vi "Tunnel position to Inside-Outside choice.vi"(7 "Default Placement":enum32{"Choice 1", "Choice 2"}(ring), 10 "Tunnel Position":enum16{"Left", "Top", "Right", "Bottom"}(ring), 11 "Action":T1=enum."Wire Properties") -> (3 "Placement":enum16{"Inside", "Outside"}(ring))   [LabVIEW 2023]
doc: "Choose default placement (inside/outisde) for a cluster element when a tunnel is selected. Bundling at the top/left of a structure assumes outisde, unbundling inside. Bundling at the bottom or right of a struncture is assumed inside, unbundling outside. This feels like the right choice in a majority of cases."
uses:
  controls/action enum.ctl
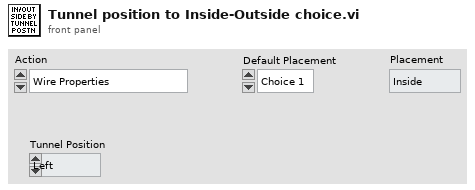
[diagram p1: front panel]
types:
  T1 = typedef "action enum.ctl" = enum16{"[NONE]", "APP_SEPARATOR", "Wire Bundle", "Wire Unbundle", "Terminal Unbundle", "Terminal Bundle", "Bundler Move Up", "Bundler Move Down", "Bundler Insert", "Bundler Remove", "Bundler Remove Unwired", "Bundler Reorder", "In Place Insert", "In Place Remove", "In Place Remove Unwired", "In Place Reorder", "Wire Properties", "Wire Method", "Terminal Properties", "Terminal Method", "Property Move Up", "Property Move Down", "Properties Insert", "Properties Remove", "Properties Remove Unwired", "Properties Reorder", "Method Change", "Class For Constant", "Class For Control", "Class For Node", "Class Name to Clipboard"}
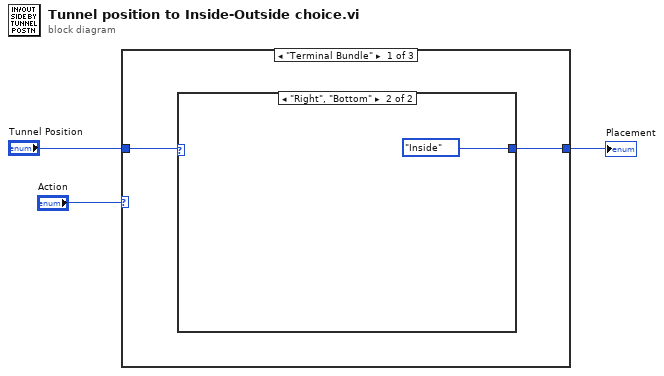
[diagram p0: block diagram]
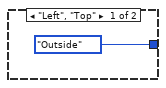
[diagram p2: hidden frame]
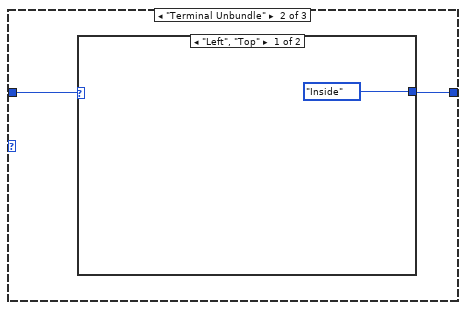
[diagram p3: hidden frame]
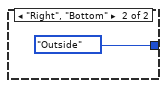
[diagram p4: hidden frame]
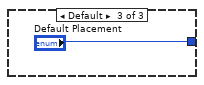
[diagram p5: hidden frame]
diagram:
  n1 = case shown="\"Terminal Bundle\"" "Action" {
    tunnel: "Tunnel Position" -> [w5 w8 _]
    tunnel: [w4 w9 "Default Placement"] -> w1
    frame "Terminal Bundle" {
      n2 = case shown="\"Right\", \"Bottom\"" w5 {
        tunnel: [enum16{"Inside", "Outside"}."Outside" ("Bundler position") enum16{"Inside", "Outside"}."Inside" ("Bundler position")] -> w4
        frame "Left", "Top" {
        }
        frame "Right", "Bottom" {
        }
      }
    }
    frame "Terminal Unbundle" {
      n3 = case shown="\"Left\", \"Top\"" w8 {
        tunnel: [enum16{"Inside", "Outside"}."Inside" ("Bundler position") enum16{"Inside", "Outside"}."Outside" ("Bundler position")] -> w9
        frame "Left", "Top" {
        }
        frame "Right", "Bottom" {
        }
      }
    }
    frame Default {
    }
  }
  "Placement" <- w1
